vi "non_FPGA_VI_v2.vi"() -> ()   [LabVIEW 2020]
uses:
  c5c29772-c0b0-45e0-ac49-cc5077cfdad3.vi
  <vilib>/Array/Sort 2D Array - Pop Stack.vi
  <vilib>/Array/Sort 2D Array - Push Stack.vi
  c5c29772-c0b0-45e0-ac49-cc5077cfdad3.vi/269d4b3b-47f5-49e3-8884-44851e4dd9d5.vi
  c5c29772-c0b0-45e0-ac49-cc5077cfdad3.vi/6d99389c-673d-4efb-bf33-19b32bcf4cf8.vi
  <vilib>/Analysis/NI_AALBase.lvlib
panel:
  out "Array 5":i32[](array[numeric])
  out "Array 4":fxp<+/-,32,21>[](array[numeric])
  out "Array 2":fxp<+/-,32,21>[](array[numeric])
  out "sorted 2D array":dbl[][](array[numeric])
  out "appended array":dbl[][](array[numeric])
  out "Array 3":i32[](array[numeric])
  out "sorted array":dbl[](array[numeric])
  out "Array":dbl[](array[numeric])
  out "uniform white noise":dbl[](array[numeric])
  out "Waveform Graph":dbl[](graph)
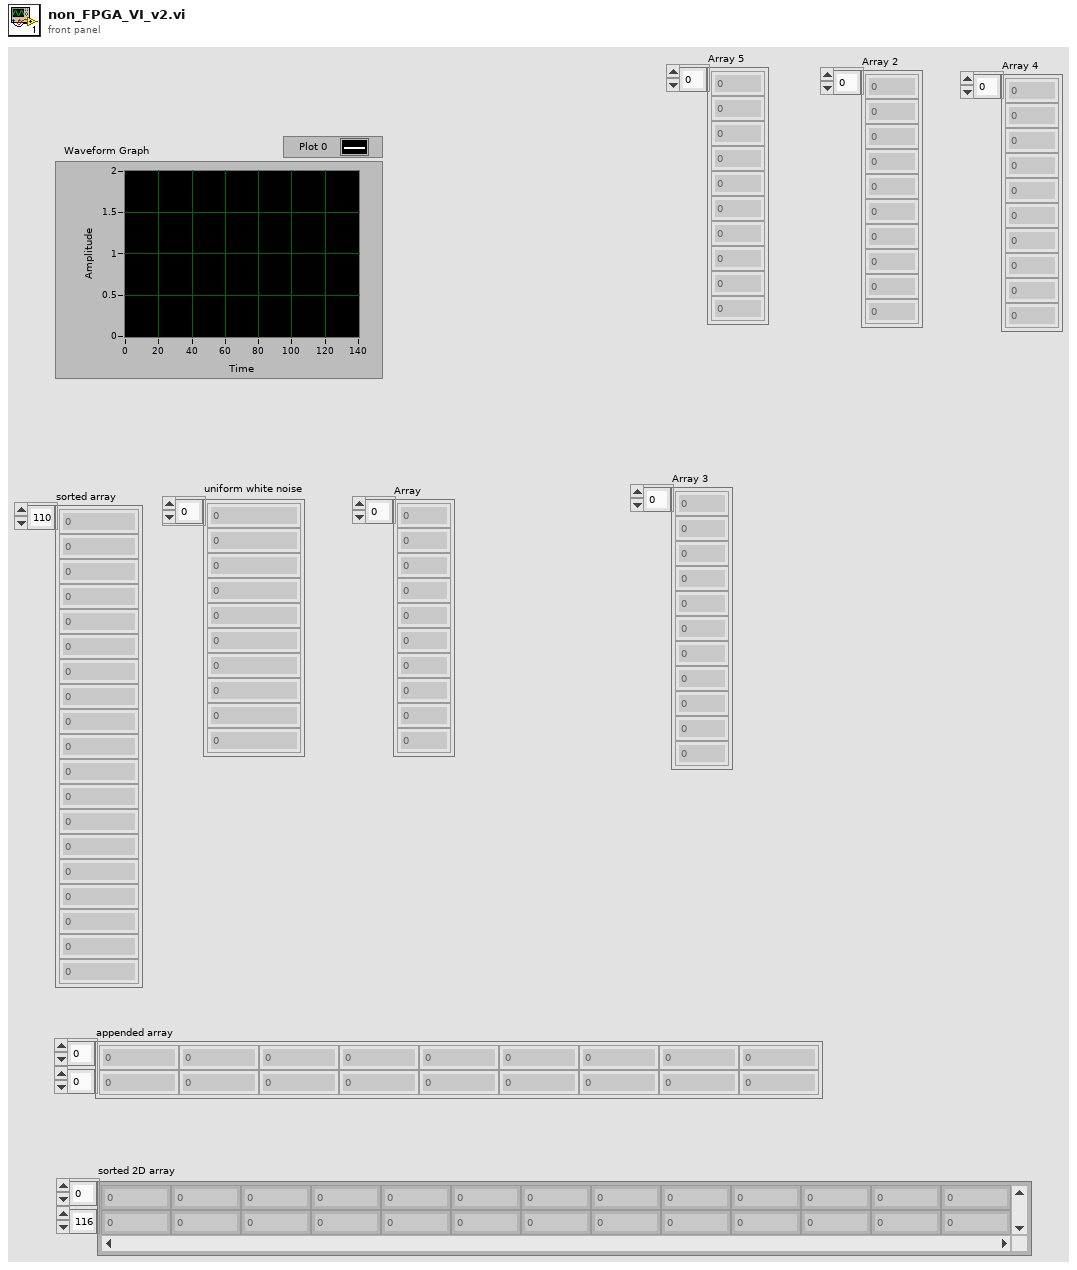
[diagram p1: front panel]
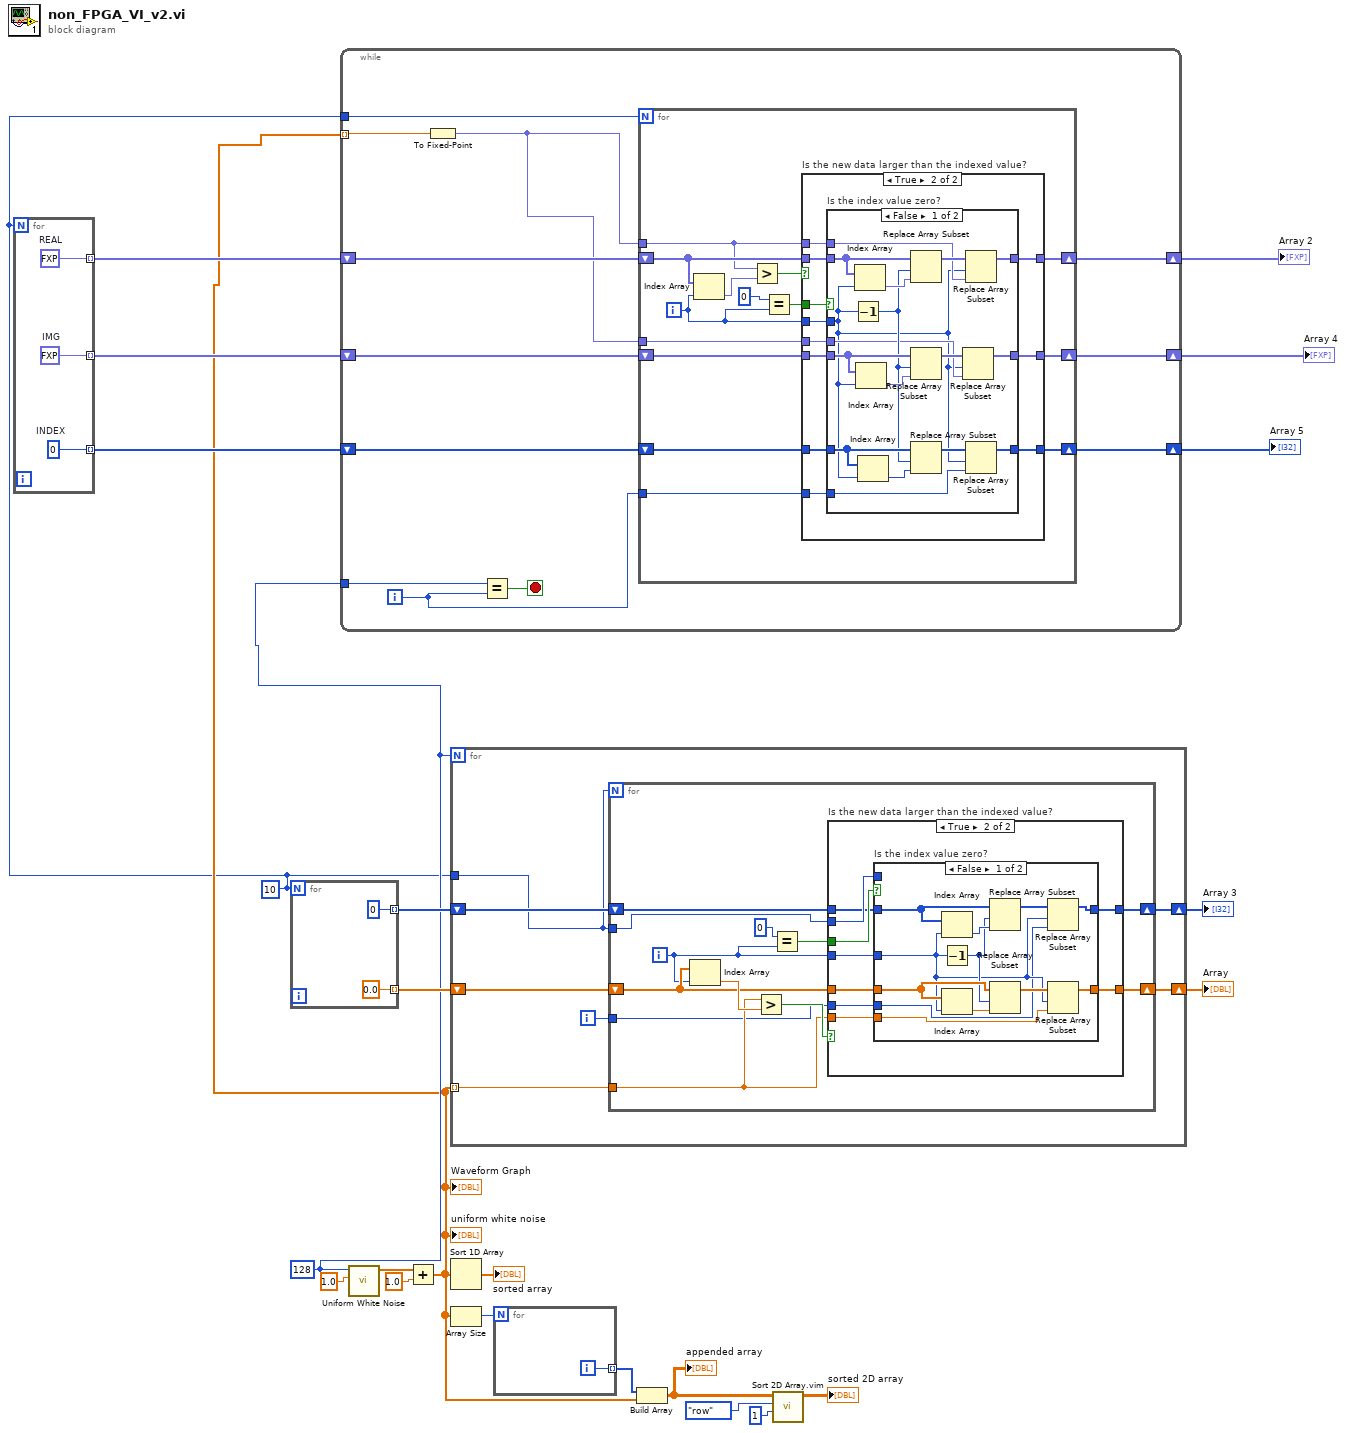
[diagram p0: block diagram]
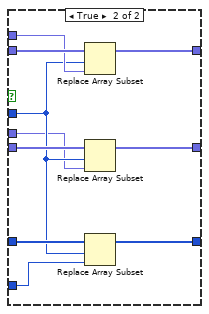
[diagram p3: hidden frame]
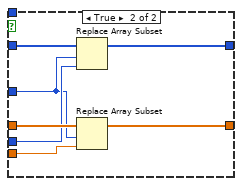
[diagram p5: hidden frame]
diagram:
  w1 = 10
  w3 = 128 ("samples")
  n1 = for {
    N: w1 -> [_]
    tunnel: [w26] -> w8 mode=indexing
    tunnel: [w25] -> w9 mode=indexing
    tunnel: [w24] -> w7 mode=indexing
    w24 = fxp<+/-,32,21> 0.0  # IMG
    w25 = 0  # INDEX
    w26 = fxp<+/-,32,21> 0.0  # REAL
  }
  n2 = for {
    N: w1 -> [_]
    tunnel: [0.0 ("amplitude")] -> w22 mode=indexing
    tunnel: [0] -> w17 mode=indexing
  }
  n3 = call <vilib>:"Uniform White Noise.vi"("amplitude"=1.0, "samples"=w3) -> ("uniform white noise"=w15:dbl[])  [unwired: 8 in, 1 out]
  n4 = Add(x=w15, y=1.0 ("amplitude")) -> (x+y=w2:dbl[])
  "Waveform Graph" <- w2
  "uniform white noise" <- w2
  n5 = while {
    shift-right: [w39] -> w5
    shift-left: w8 -> [w40]
    shift-right: [w38] -> w6
    shift-left: w9 -> [w37]
    tunnel: w3 -> [w35]
    shift-right: [w33] -> w4
    shift-left: w7 -> [w32]
    tunnel: w2 -> [w31] mode=indexing
    tunnel: w1 -> [w29]
    i -> [w36]
    stop <- w34 stop-if-true
    n6 = To Fixed-Point(number=w31) -> (fixed-point=w30:fxp<+/-,32,16>)  [unwired: 1 in]
    n7 = Equal?(x=w35, y=w36) -> (x = y?=w34:bool)
    n8 = for {
      N: w29 -> [_]
      tunnel: w30 -> [w51]
      shift-right: [w50] -> w39
      shift-left: w40 -> [w52]
      tunnel: w36 -> [w48]
      shift-right: [w46] -> w38
      shift-left: w37 -> [w47]
      shift-right: [w43] -> w33
      shift-left: w32 -> [w42]
      tunnel: w30 -> [w41]
      i -> [w49]
      n9 = Index Array(array=w52, index=w49) -> (element=w54:fxp<+/-,32,21>)
      n10 = Greater?(x=w51, y=w54) -> (0:w53:bool)
      n11 = Equal?(x=0, y=w49) -> (x = y?=w44:bool)
      n12 = case "Is the new data larger than the indexed value?" shown="True" w53 {
        tunnel: w52 -> [w57 w67]
        tunnel: w44 -> [_ w68]
        tunnel: w51 -> [_ w66]
        tunnel: w49 -> [_ w65]
        tunnel: [w57 w64] -> w50
        tunnel: w48 -> [_ w63]
        tunnel: w47 -> [w56 w62]
        tunnel: [w56 w61] -> w46
        tunnel: [w55 w60] -> w43
        tunnel: w42 -> [w55 w59]
        tunnel: w41 -> [_ w58]
        frame False {
        }
        frame True {
          n13 = case "Is the index value zero?" shown="False" w68 {
            tunnel: w67 -> [w85 w95]
            tunnel: w66 -> [w82 w94]
            tunnel: w65 -> [w69 w88]
            tunnel: [w81 w93] -> w64
            tunnel: w63 -> [w76 w92]
            tunnel: w62 -> [w78 w91]
            tunnel: [w77 w90] -> w61
            tunnel: [w71 w86] -> w60
            tunnel: w59 -> [w75 w89]
            tunnel: w58 -> [w70 w87]
            frame False {
              n14 = Decrement(x=w69) -> (x-1=w73:i32)
              n15 = Index Array(array=w85, index=w69) -> (element=w84:fxp<+/-,32,21>)
              n16 = Index Array(array=w75, index=w69) -> (element=w74:fxp<+/-,32,21>)
              n17 = Index Array(array=w78, index=w69) -> (element=w80:i32)
              n18 = Replace Array Subset(array=w85, new element=w84, index=w73) -> (w83:fxp<+/-,32,21>[])
              n19 = Replace Array Subset(array=w75, new element=w74, index=w73) -> (w72:fxp<+/-,32,21>[])
              n20 = Replace Array Subset(array=w78, new element=w80, index=w73) -> (w79:i32[])
              n21 = Replace Array Subset(array=w72, new element=w70, index=w69) -> (w71:fxp<+/-,32,21>[])
              n22 = Replace Array Subset(array=w83, new element=w82, index=w69) -> (w81:fxp<+/-,32,21>[])
              n23 = Replace Array Subset(array=w79, new element=w76, index=w69) -> (w77:i32[])
            }
            frame True {
              n24 = Replace Array Subset(array=w95, new element=w94, index=w88) -> (w93:fxp<+/-,32,21>[])
              n25 = Replace Array Subset(array=w89, new element=w87, index=w88) -> (w86:fxp<+/-,32,21>[])
              n26 = Replace Array Subset(array=w91, new element=w92, index=w88) -> (w90:i32[])
            }
          }
        }
      }
    }
  }
  "Array 2" <- w5
  "Array 4" <- w4
  "Array 5" <- w6
  n27 = for {
    N: w3 -> [_]
    tunnel: w2 -> [w102] mode=indexing
    shift-right: [w100] -> w21
    shift-left: w22 -> [w101]
    shift-right: [w98] -> w18
    shift-left: w17 -> [w97]
    tunnel: w1 -> [w96]
    i -> [w99]
    n28 = for {
      N: w96 -> [_]
      tunnel: w102 -> [w109]
      tunnel: w96 -> [w107]
      shift-right: [w108] -> w100
      shift-left: w101 -> [w112]
      tunnel: w99 -> [w105]
      shift-right: [w103] -> w98
      shift-left: w97 -> [w104]
      i -> [w106]
      n29 = Index Array(array=w112, index=w106) -> (element=w114:dbl)
      n30 = Greater?(x=w109, y=w114) -> (0:w113:bool)
      n31 = Equal?(x=0, y=w106) -> (x = y?=w110:bool)
      n32 = case "Is the new data larger than the indexed value?" shown="True" w113 {
        tunnel: w112 -> [w116 w124]
        tunnel: w110 -> [_ w125]
        tunnel: w107 -> [_ w123]
        tunnel: w109 -> [_ w122]
        tunnel: w106 -> [_ w121]
        tunnel: [w116 w120] -> w108
        tunnel: w105 -> [_ w119]
        tunnel: w104 -> [w115 w118]
        tunnel: [w115 w117] -> w103
        frame False {
        }
        frame True {
          n33 = case "Is the index value zero?" shown="False" w125 {
            tunnel: w124 -> [w137 w144]
            tunnel: w123 -> [_ _]
            tunnel: w122 -> [w134 w143]
            tunnel: w121 -> [w127 w140]
            tunnel: [w133 w142] -> w120
            tunnel: w119 -> [w126 w141]
            tunnel: w118 -> [w130 w139]
            tunnel: [w129 w138] -> w117
            frame False {
              n34 = Index Array(array=w130, index=w127) -> (element=w132:i32)
              n35 = Decrement(x=w127) -> (x-1=w128:i32)
              n36 = Index Array(array=w137, index=w127) -> (element=w136:dbl)
              n37 = Replace Array Subset(array=w130, new element=w132, index=w128) -> (w131:i32[])
              n38 = Replace Array Subset(array=w137, new element=w136, index=w128) -> (w135:dbl[])
              n39 = Replace Array Subset(array=w131, new element=w126, index=w127) -> (w129:i32[])
              n40 = Replace Array Subset(array=w135, new element=w134, index=w127) -> (w133:dbl[])
            }
            frame True {
              n41 = Replace Array Subset(array=w139, new element=w141, index=w140) -> (w138:i32[])
              n42 = Replace Array Subset(array=w144, new element=w143, index=w140) -> (w142:dbl[])
            }
          }
        }
      }
    }
  }
  "Array" <- w21
  "Array 3" <- w18
  n43 = Sort 1D Array(array=w2) -> (sorted array=→"sorted array":dbl[])
  n44 = Array Size(array=w2) -> (size(s)=w16:i32)
  n45 = for {
    N: w16 -> [_]
    tunnel: [w145] -> w14 mode=indexing
    i -> [w145]
  }
  n46 = Build Array(w14, w2) -> (w13:dbl[][])
  "appended array" <- w13
  n47 = call "Sort 2D Array.vim"("index"=1, "dimension to index (column)"=enum16{"column", "row"}."row", "2D array"=w13) -> ("sorted 2D array"=→"sorted 2D array":dbl[][])  [unwired: 7 in, 1 out]
